vi "Open CAN Session.vi"(8 "error in":errorcluster) -> (0 "error out":errorcluster, 3 "CAN Session":T1)   [LabVIEW 2016]
doc: "This VI starts the CAN communication thread using VI server and it returns a refnum to that thread."
uses:
  Low Level VIs/Typedefs/CAN Refnum.ctl
  Low Level VIs/Typedefs/CAN Session Pointer.ctl
  Low Level VIs/Typedefs/CAN Communication References.ctl
  Low Level VIs/Typedefs/kill process notifier array.ctl
  Low Level VIs/Typedefs/Write Queue.ctl
  Low Level VIs/Typedefs/FPGA CAN Frame Cluster.ctl
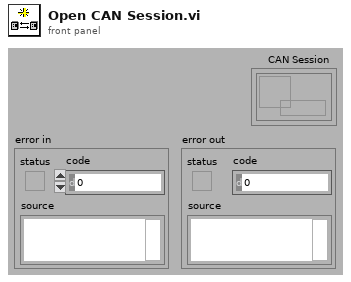
[diagram p1: front panel]
types:
  T1 = typedef "CAN Refnum.ctl" = refnum<k1>
  T2 = typedef "Write Queue.ctl" = refnum<queue>
  T3 = typedef "FPGA CAN Frame Cluster.ctl" = cluster{"Timestamp":u64, "Identifier":u32, "Type":u8, "InfoA":u8, "InfoB":u8, "DataLength":u8, "Data":u8[]}
  T4 = typedef "CAN Communication References.ctl" = cluster{"kill process notifier array":T5, "Write Queue":T2, "New Frame Notifier":refnum<notifier>, "Read Queue Array":T2[]}
  T5 = typedef "kill process notifier array.ctl" = refnum<notifier>[]
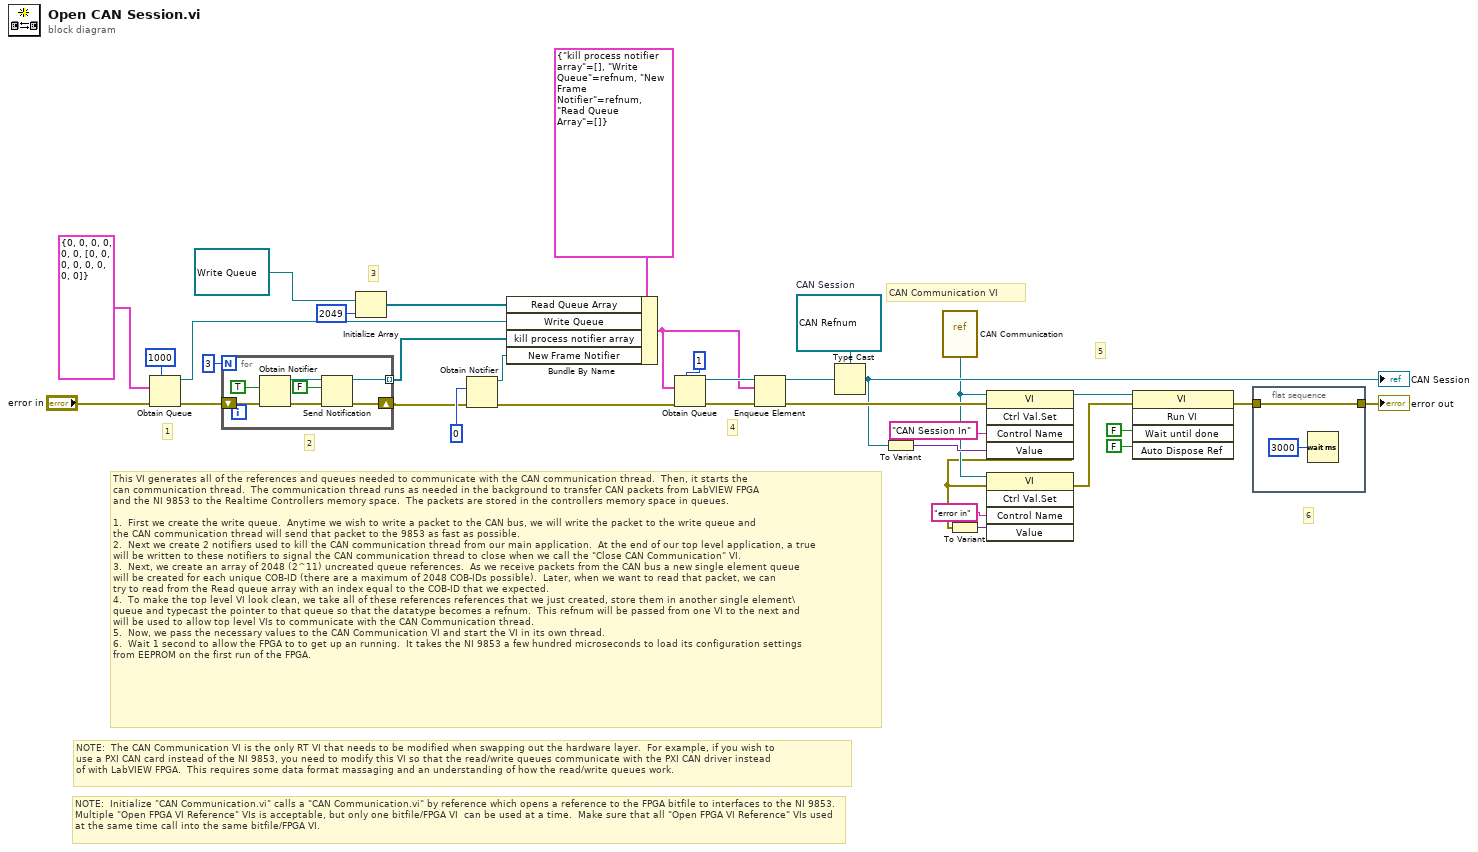
[diagram p0: block diagram]
diagram:
  w32 = T1 refnum  # CAN Session
  # "6"
  # "NOTE:  Initialize \"CAN Communication.vi\" calls a \"CAN Communication.vi\" by reference which opens a reference to the FPGA bitfile to interfaces to the NI 9853.  Multiple \"Open FPGA VI Reference\" VIs is acceptable, but only one bitfile/FPGA VI  can be used at a time.  Make sure that all \"Open FPGA VI Reference\" VIs used at the same time call into the same bitfile/FPGA VI."
  # "NOTE:  The CAN Communication VI is the only RT VI that needs to be modified when swapping out the hardware layer.  For example, if you wish to\nuse a PXI CAN card instead of the NI 9853, you need to modify this VI so that the read/write queues communicate with the PXI CAN driver instead\nof with LabVIEW FPGA.  This requires some data format massaging and an understanding of how the read/write queues work."
  # "CAN Communication VI"
  # "5"
  # "4"
  # "2"
  # "This VI generates all of the references and queues needed to communicate with the CAN communication thread.  Then, it starts the\ncan communication thread.  The communication thread runs as needed in the background to transfer CAN packets from LabVIEW FPGA\nand the NI 9853 to the Realtime Controllers memory space.  The packets are stored in the controllers memory space in queues.\n\n1.  First we create the write queue.  Anytime we wish to write a packet to the CAN bus, we will write the packet to the write queue and\nthe CAN communication thread will send that packet to the 9853 as fast as possible.\n2.  Next we create 2 notifiers used to kill the CAN communication thread from our main application.  At the end of our top level application, a true\nwill be written to these notifiers to signal the CAN communication thread to close when we call the \"Close CAN Communication\" VI.\n3.  Next, we create an array of 2048 (2^11) uncreated queue references.  As we receive packets from the CAN bus a new single element queue\nwill be created for each unique COB-ID (there are a maximum of 2048 COB-IDs possible).  Later, when we want to read that packet, we can\ntry to read from the Read queue array with an index equal to the COB-ID that we expected.\n4.  To make the top level VI look clean, we take all of these references references that we just created, store them in another single element\\\nqueue and typecast the pointer to that queue so that the datatype becomes a refnum.  This refnum will be passed from one VI to the next and\nwill be used to allow top level VIs to communicate with the CAN Communication thread.\n5.  Now, we pass the necessary values to the CAN Communication VI and start the VI in its own thread.\n6.  Wait 1 second to allow the FPGA to to get up an running.  It takes the NI 9853 a few hundred microseconds to load its configuration settings\nfrom EEPROM on the first run of the FPGA."
  # "3"
  # "1"
  n1 = Obtain Queue(max queue size (-1, unlimited)=1000, element data type=T3 {"Timestamp"=0, "Identifier"=0, "Type"=0, "InfoA"=0, "InfoB"=0, "DataLength"=0, "Data"=[0, 0, 0, 0, 0, 0, 0, 0]} ("CAN Frame"), error in (no error)="error in") -> (queue out=w12:refnum<queue>, error out=w27:errorcluster)  [unwired: 1 in, 2 out]
  n2 = for {
    N: 3 -> [_]
    tunnel: [w37] -> w15 mode=indexing
    shift-right: [w36] -> w4
    shift-left: w27 -> [w42]
    n3 = Obtain Notifier(notification data type=TRUE, error in (no error)=w42) -> (notifier out=w39:refnum<notifier>, error out=w40:errorcluster)  [unwired: 1 in, 2 out]
    n4 = Send Notification(notification=FALSE, notifier=w39, error in (no error)=w40) -> (notifier out=w37:refnum<notifier>, error out=w36:errorcluster)
  }
  n5 = Initialize Array(T2 refnum ("Write Queue"), 2049 ("dimension size")) -> (w2:T2[])
  n6 = Obtain Notifier(notification data type=0, error in (no error)=w4) -> (notifier out=w3:refnum<notifier>, error out=w6:errorcluster)  [unwired: 2 in, 1 out]
  n7 = Bundle By Name(cluster=T4 {"kill process notifier array"=[], "Write Queue"=refnum, "New Frame Notifier"=refnum, "Read Queue Array"=[]} ("CAN Communication References"), "Read Queue Array"=w2, "Write Queue"=w12, "kill process notifier array"=w15, "New Frame Notifier"=w3) -> (w11:T4)
  n8 = Obtain Queue(max queue size (-1, unlimited)=1, element data type=w11, error in (no error)=w6) -> (queue out=w29:refnum<queue>, error out=w30:errorcluster)  [unwired: 1 in, 2 out]
  n9 = Enqueue Element(queue=w29, element=w11, error in (no error)=w30) -> (queue out=w28:refnum<queue>, error out=w23:errorcluster)  [unwired: 2 out]
  n10 = Type Cast(type=w32, x=w28) -> (*(type *) &x=w16:T1)
  "CAN Session" <- w16
  n11 = To Variant(anything=w16) -> (Variant=w22:variant)
  n12 = vi-ref "CAN Communication.vi"() -> (w10:refnum<vi>)
  n13 = invoke class="VI" method="Ctrl Val.Set"(reference=w10, error in=w23, "Control Name"="CAN Session In", "Value"=w22) -> (reference out=w18:refnum<vi>, error out=w9:errorcluster)  [unwired: 1 in, 3 out]
  n14 = To Variant(anything=w9) -> (Variant=w21:variant)
  n15 = invoke class="VI" method="Ctrl Val.Set"(reference=w10, error in=w9, "Control Name"="error in", "Value"=w21) -> (error out=w17:errorcluster)  [unwired: 1 in, 4 out]
  n16 = invoke class="VI" method="Run VI"(reference=w18, error in=w17, "Wait until done"=FALSE ("Wait Until Done"), "Auto Dispose Ref"=FALSE ("Auto Dispose Reference")) -> (error out=w8:errorcluster)  [unwired: 1 in, 4 out]
  n17 = flat-sequence {
    tunnel: w8 -> [w44]
    tunnel: [w44] -> w7
    frame #0 {
      n18 = Wait (ms)(milliseconds to wait=u32 3000) -> ()  [unwired: 1 out]
    }
  }
  "error out" <- w7
